vi "LinearBearingControl.vi"() -> ()   [LabVIEW 2012]
uses:
  stressTestTypeDef.ctl
  <vilib>/Utility/error.llb/DialogType.ctl
  allStatesTypeDef.ctl
  <vilib>/Utility/file.llb/Write To Spreadsheet File (DBL).vi
panel:
  out "mm/s (timed)":dbl
  in  "Direction":bool
  in  "Only Move Lin":bool
  out "writing data":bool
  out "stop sys":bool
  out "udp error out":errorcluster
  out "Voltages":dbl[][](array[numeric])
  in  "Start System":bool
  in  "Auto Bias":bool=TRUE
  in  "Unbias":bool
  in  "Bias":bool
  in  "Collect Data":bool=TRUE
  out "Measurement":dbl[][](graph) caption="F/T Data"
  out "Bias Vector":dbl[](array[numeric])
  in  "Timing parameters":T1={"Sample Rate"=1000.0, "Samples to Read"=100}
  in  "Transform":T2
  in  "Channel Parameters":T3={"First Channel"=1, "Number of Channels"=6, "DAQ Card"="Dev2", "Maximum Value"=10.0, "Minimum Value"=-10.0}
  in  "Sensor Parameters":T4={"Calibration File"=path "D:/ArduinoSmarticle/entangledSmarticle/FT21164.cal", "Force Units"="N", "Torque Units"="N-mm"}
  out "filenameOut":string
  in  "Optitrack Parameters":T5={"Optitrack IP"="130.207.141.229", "Optitrack Port"=1520, "timeout (sec)"=80}
  out "Data Output File":path
  in  "Output Folder":path=path "D:/ArduinoSmarticle/entangledSmarticle/Results"
  in  "Program Parameters":T7={"v"=1, "Iters"=2, "Speed"=49, "Delay"=4, "H"=10.5, "SD"=240, "Name"="SS", "Type"=enum."OFF"} {"Speed" min=0 max=49}
  out "strain %":dbl
  out "FT error out":errorcluster
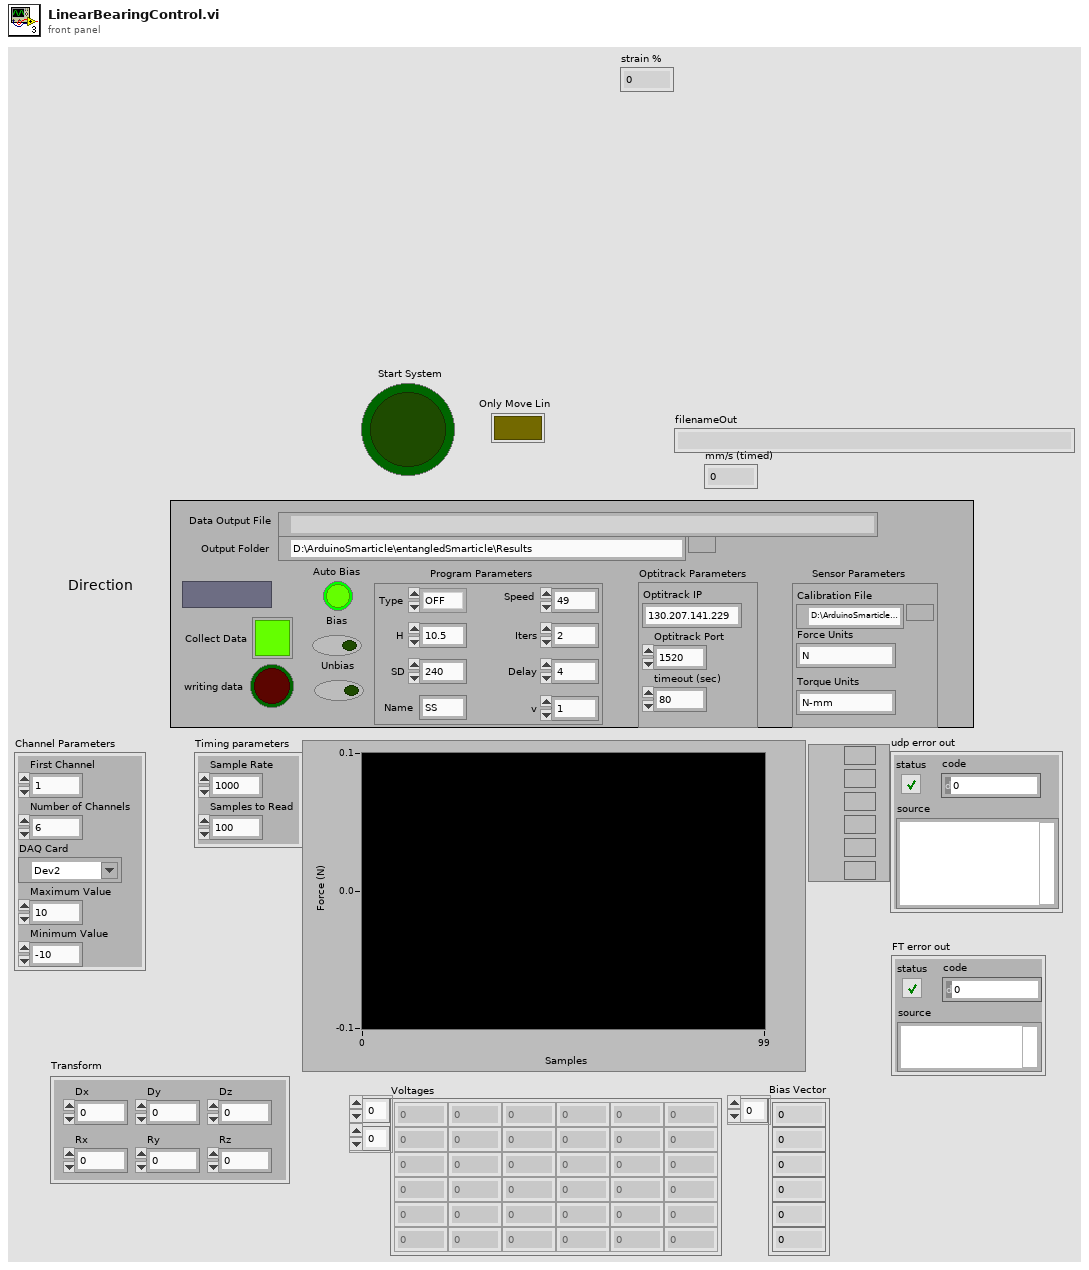
[diagram p1: front panel]
types:
  T1 = cluster{"Sample Rate":dbl, "Samples to Read":i32}
  T2 = cluster{"Dx":dbl, "Dy":dbl, "Dz":dbl, "Rx":dbl, "Ry":dbl, "Rz":dbl}
  T3 = cluster{"First Channel":i16, "Number of Channels":i16, "DAQ Card":tag, "Maximum Value":dbl, "Minimum Value":dbl}
  T4 = cluster{"Calibration File":path, "Force Units":string, "Torque Units":string}
  T5 = cluster{"Optitrack IP":string, "Optitrack Port":u16, "timeout (sec)":i32}
  T6 = typedef "stressTestTypeDef.ctl" = enum16{"OFF", "ON", "EXTEND", "SPRING", "FRACT ON", "SAC", "FRACT SAC"}
  T7 = cluster{"v":i32, "Iters":i32, "Speed":i32, "Delay":i32, "H":dbl, "SD":i32, "Name":string, "Type":T6}
  T8 = typedef "DialogType.ctl" = u16
  T9 = cluster{"SD":i32, "Delay":i32, "Speed":i32, "Iters":i32, "Type":T6}
  T10 = typedef "allStatesTypeDef.ctl" = enum16{"open udp", "start record", "recording", "move linear actuator", "end record", "close udp", "end"}
  T11 = cluster{"distance mm":i32, "Direction":bool, "speed (mm/s)":i32}
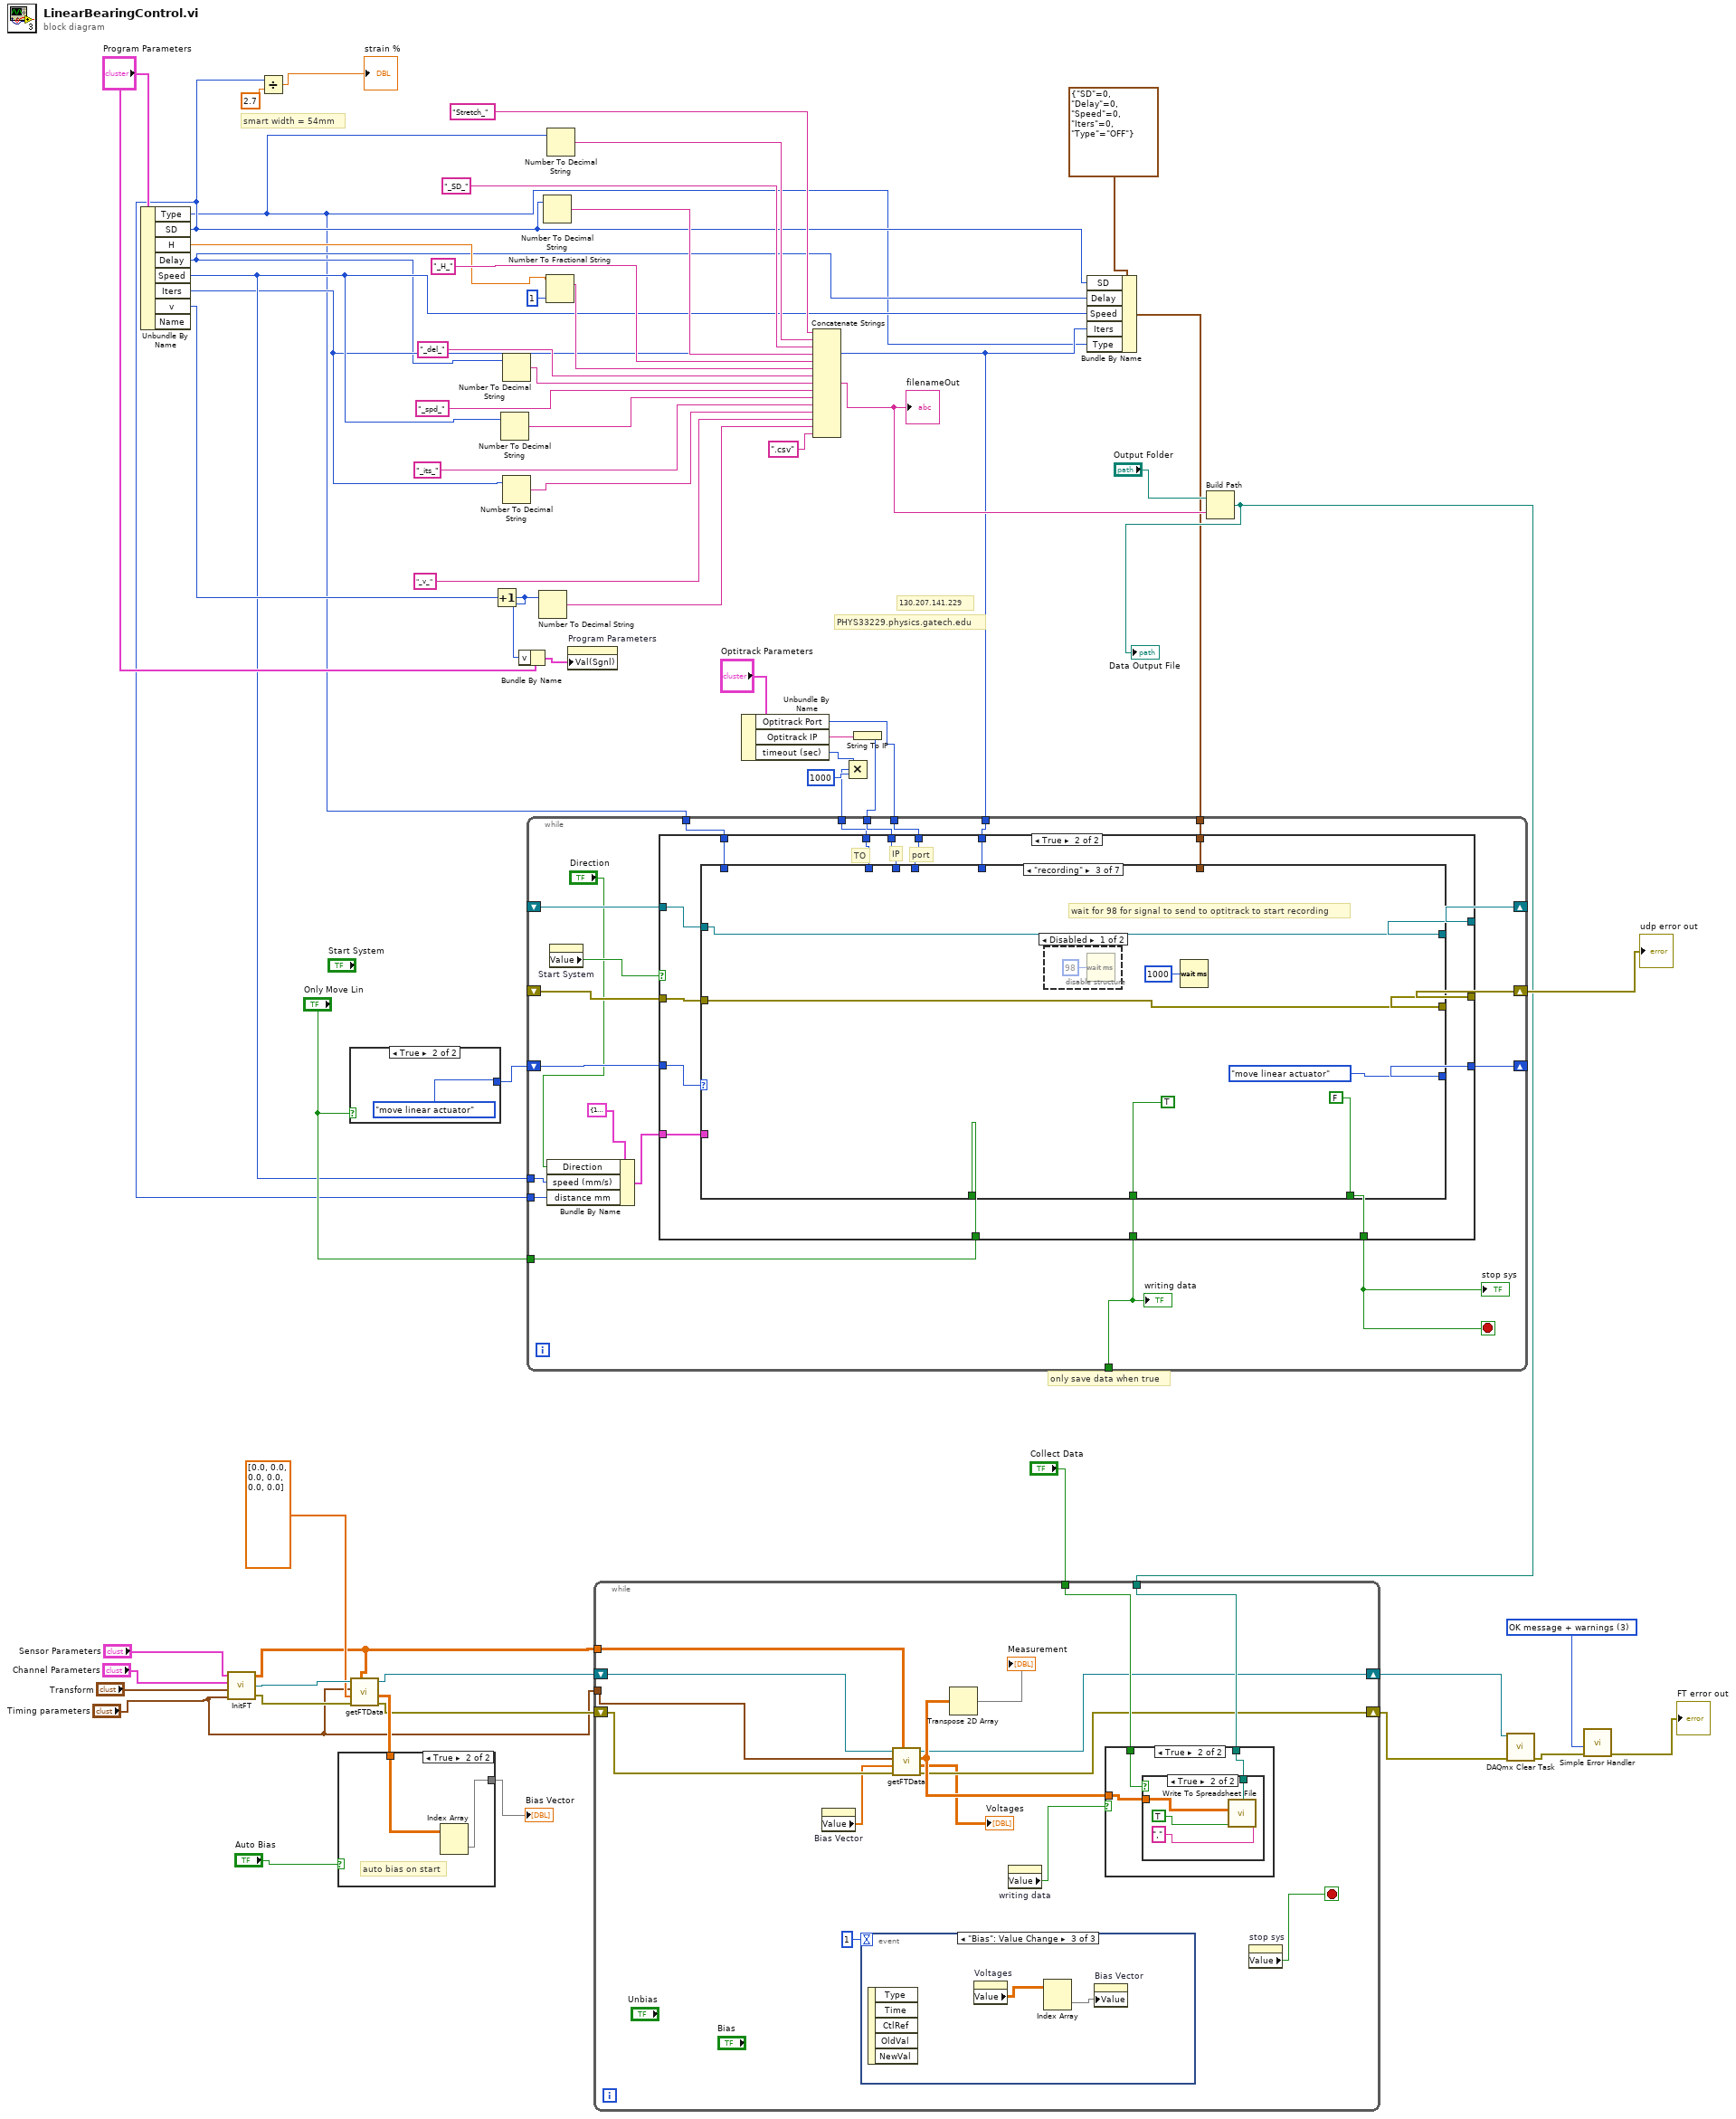
[diagram p0: block diagram]
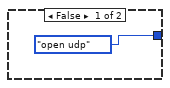
[diagram p2: hidden frame]
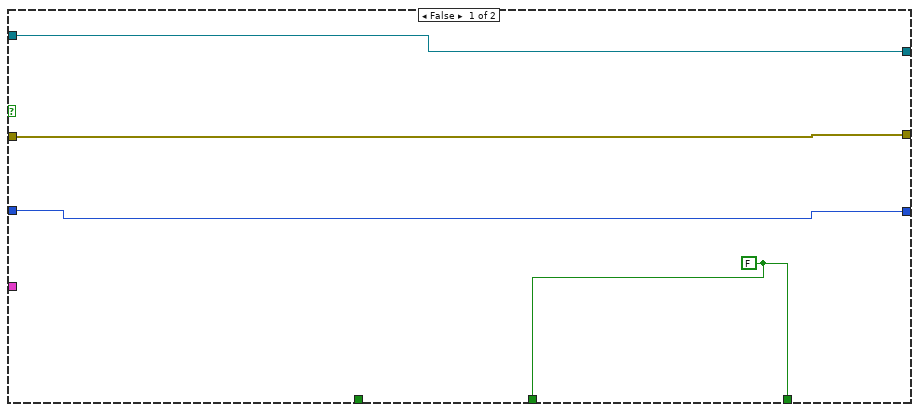
[diagram p3: hidden frame]
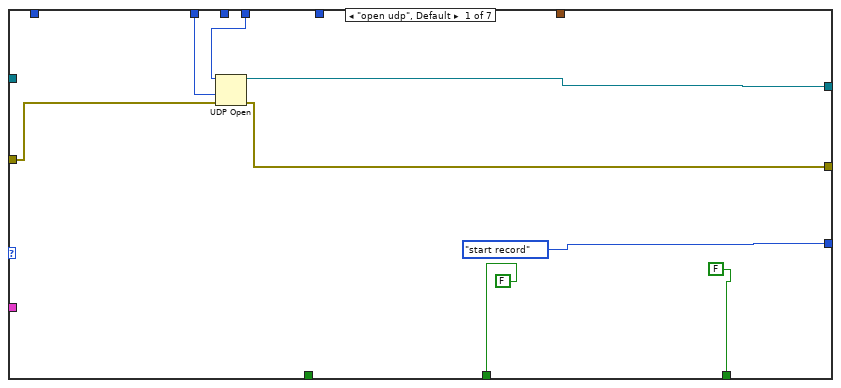
[diagram p4: hidden frame]
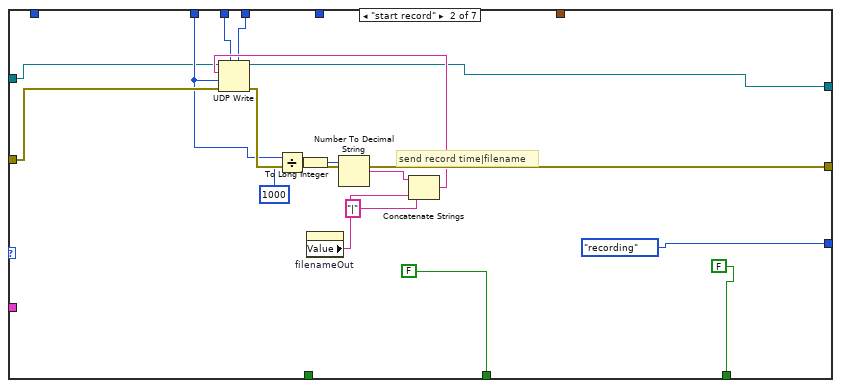
[diagram p5: hidden frame]
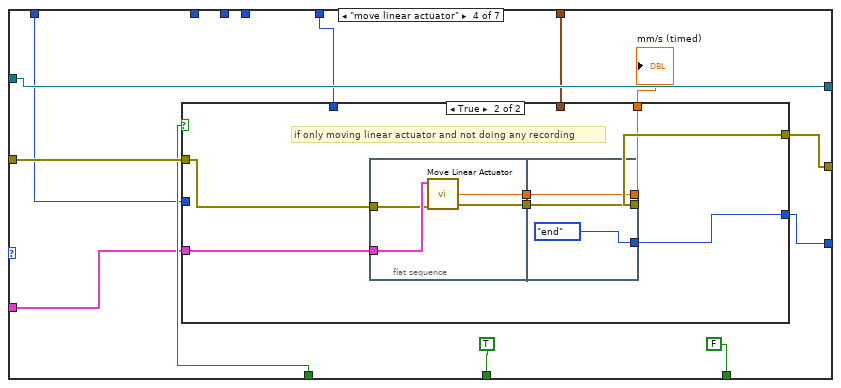
[diagram p7: hidden frame]
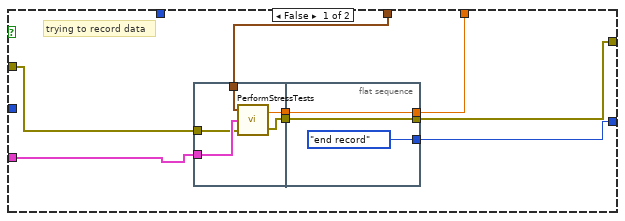
[diagram p8: hidden frame]
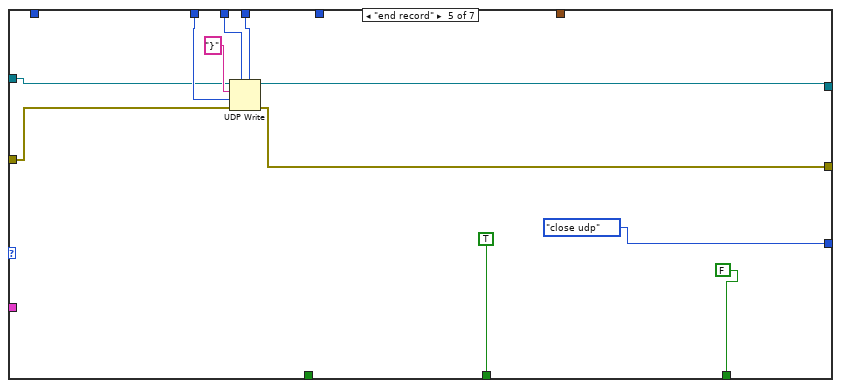
[diagram p9: hidden frame]
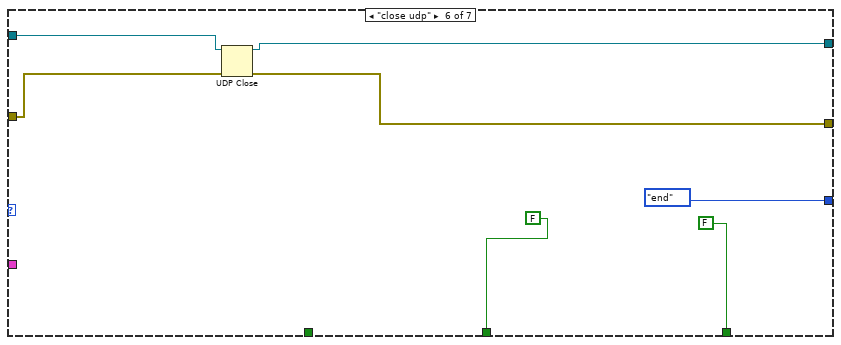
[diagram p10: hidden frame]
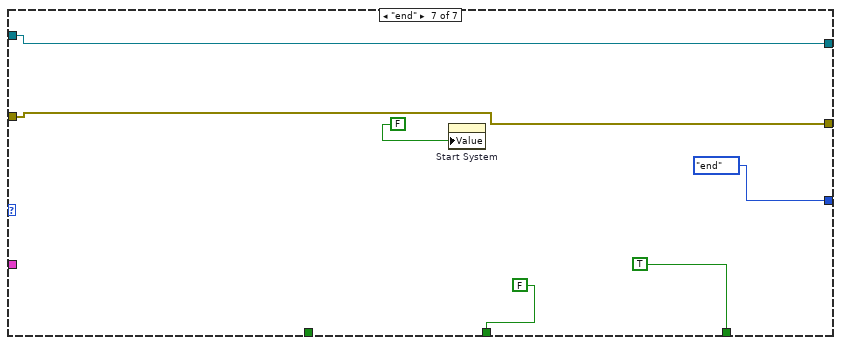
[diagram p11: hidden frame]
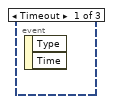
[diagram p12: hidden frame]
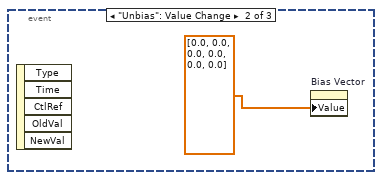
[diagram p13: hidden frame]
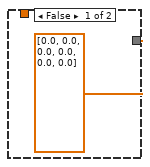
[diagram p16: hidden frame]
diagram:
  w27 = T8 3 items=["no dialog", "OK message", "continue or stop message", "OK message + warnings", "continue/stop + warnings"] ("type of dialog (OK msg:1)")
  # "only save data when true"
  # "smart width = 54mm"
  # "PHYS33229.physics.gatech.edu"
  # "130.207.141.229"
  n1 = Unbundle By Name("Program Parameters") -> ("Type"=w2:T6, "SD"=w5:i32, "H"=w42:dbl, "Delay"=w3:i32, "Speed"=w6:i32, "Iters"=w4:i32, "v"=w43:i32)  [unwired: 1 out]
  n2 = call "InitFT.vi"("Timing parameters"="Timing parameters", "Transform"="Transform", "Channel Parameters"="Channel Parameters", "Sensor Parameters"="Sensor Parameters") -> ("error out"=w23:errorcluster, "task out"=w24:refnum<k21>, "Calibration Matrix"=w18:dbl[][])
  n3 = Divide(x=w5, y=2.7) -> (x/y=→"strain %":dbl)
  n4 = case shown="True" "Only Move Lin" {
    tunnel: [allStatesTypeDef."open udp" allStatesTypeDef."move linear actuator"] -> w62
    frame False {
    }
    frame True {
    }
  }
  n5 = call "getFTData.vi"("Transformed Calibration Matrix"=w18, "error in"=w23, "Bias Vector"=dbl[] [0.0, 0.0, 0.0, 0.0, 0.0, 0.0], "Timing parameters"="Timing parameters", "task in"=w24) -> ("error out"=w16:errorcluster, "Voltages"=w21:dbl[][], "task out 2"=w17:refnum<k21>)  [unwired: 1 out]
  n6 = case shown="True" "Auto Bias" {
    tunnel: w21 -> [_ w67]
    tunnel: [dbl[] [0.0, 0.0, 0.0, 0.0, 0.0, 0.0] w66] -> w14
    frame False {
    }
    frame True {
      # "auto bias on start"
      n7 = Index Array(array=w67) -> (element=w66:dbl[])  [unwired: 2 in]
    }
  }
  "Bias Vector" <- w14
  n8 = Increment(x=w43) -> (x+1=w44:i32)
  n9 = Number To Decimal String(number=w6) -> (decimal integer string=w48:string)  [unwired: 1 in]
  n10 = Number To Decimal String(number=w3) -> (decimal integer string=w54:string)  [unwired: 1 in]
  n11 = Number To Decimal String(number=w4) -> (decimal integer string=w46:string)  [unwired: 1 in]
  n12 = Bundle By Name(cluster="Program Parameters", "v"=w44) -> (w38:T7)
  n13 = Number To Decimal String(number=w44) -> (decimal integer string=w50:string)  [unwired: 1 in]
  n14 = Number To Decimal String(number=w5) -> (decimal integer string=w57:string)  [unwired: 1 in]
  n15 = Number To Fractional String(number=w42, precision (6)=i16 1) -> (F-format string=w53:string)  [unwired: 2 in]
  n16 = Number To Decimal String(number=w2) -> (decimal integer string=w59:string)  [unwired: 1 in]
  n17 = property on="Program Parameters" class="Clust (strict)"("Val(Sgnl)"=w38) -> ()  [unwired: 2 in, 2 out]
  n18 = Unbundle By Name("Optitrack Parameters") -> ("Optitrack Port"=w36:u16, "Optitrack IP"=w35:string, "timeout (sec)"=w33:i32)
  n19 = Concatenate Strings("Stretch_", w59, "_SD_", w57, "_H_", w53, "_del_", w54, "_spd_", w48, "_its_", w46, "_v_", w50, ".csv") -> (w8:string)
  "filenameOut" <- w8
  n20 = Multiply(x=w33, y=1000) -> (x*y=w31:i32)
  n21 = String To IP(1:w35) -> (0:w34:u32)
  n22 = Bundle By Name(cluster=T9 {"SD"=0, "Delay"=0, "Speed"=0, "Iters"=0, "Type"=enum."OFF"}, "SD"=w5, "Delay"=w3, "Speed"=w6, "Iters"=w4, "Type"=w2) -> (w1:T9)
  n23 = while {
    shift-right: [w88] -> w11
    shift-left: _ -> [w87]
    shift-right: [w85] -> _
    shift-left: w62 -> [w86]
    tunnel: w36 -> [w83]
    tunnel: w34 -> [w84]
    tunnel: w31 -> [w82]
    shift-right: [w81] -> _
    shift-left: _ -> [w80]
    tunnel: [w79] -> _
    tunnel: "Only Move Lin" -> [w76]
    tunnel: w6 -> [w73]
    tunnel: w5 -> [w72]
    tunnel: w2 -> [w70]
    tunnel: w4 -> [w69]
    tunnel: w1 -> [w68]
    stop <- w78 stop-if-true
    n24 = Bundle By Name(cluster=T11 {"distance mm"=100, "Direction"=FALSE, "speed (mm/s)"=18} ("linear actuator info"), "Direction"="Direction", "speed (mm/s)"=w73, "distance mm"=w72) -> (w75:T11)
    n25 = property on="Start System" class="Bool (strict)"() -> ("Value"=w77:bool)  [unwired: 2 in, 2 out]
    n26 = case shown="True" w77 {
      tunnel: [w89 w108] -> w88
      tunnel: w87 -> [w89 w107]
      tunnel: w86 -> [w92 w106]
      tunnel: [w92 w105] -> w85
      tunnel: w84 -> [_ w104]
      tunnel: w83 -> [_ w97]
      tunnel: w82 -> [_ w103]
      tunnel: [w90 w102] -> w81
      tunnel: w80 -> [w90 w101]
      tunnel: [w91 w100] -> w79
      tunnel: [w91 w99] -> w78
      tunnel: w76 -> [_ w98]
      tunnel: w75 -> [_ w96]
      tunnel: w70 -> [_ w95]
      tunnel: w69 -> [_ w94]
      tunnel: w68 -> [_ w93]
      frame False {
        w91 = FALSE
      }
      frame True {
        # "IP"
        # "TO"
        # "port"
        n27 = case shown="\"recording\"" w106 {
          tunnel: w103 -> [w113 w125 _ _ w189 _ _]
          tunnel: w107 -> [w114 w131 w135 w148 w193 w199 w201]
          tunnel: [w115 w132 w135 w147 w192 w200 w201] -> w108
          tunnel: [allStatesTypeDef."start record" allStatesTypeDef."recording" allStatesTypeDef."move linear actuator" w150 allStatesTypeDef."close udp" allStatesTypeDef."end" allStatesTypeDef."end"] -> w105
          tunnel: [FALSE FALSE FALSE FALSE FALSE FALSE TRUE] -> w99
          tunnel: w104 -> [_ w118 _ _ w183 _ _]
          tunnel: [w112 w121 w136 w149 w187 w198 w206] -> w102
          tunnel: w101 -> [_ w122 w136 w149 w186 w194 w206]
          tunnel: [FALSE FALSE TRUE TRUE TRUE FALSE FALSE] -> w100
          tunnel: w98 -> [_ _ _ w146 _ _ _]
          tunnel: w97 -> [w109 w117 _ _ w184 _ _]
          tunnel: w96 -> [_ _ _ w145 _ _ _]
          tunnel: w95 -> [_ _ _ w142 _ _ _]
          tunnel: w94 -> [_ _ _ w143 _ _ _]
          tunnel: w93 -> [_ _ _ w141 _ _ _]
          frame "open udp", Default {
            n28 = UDP Open(8:w114, 9:w113, 11:w109) -> (port=w112:refnum<k16>, 0:w115:errorcluster)  [unwired: 2 in, 1 out]
          }
          frame "start record" {
            # "send record time|filename"
            n29 = Divide(x=w125, y=1000) -> (x/y=w124:dbl)
            n30 = To Long Integer(number=w124) -> (32bit integer=w123:i32)
            n31 = property on="filenameOut" class="Str"() -> ("Value"=w129:string)  [unwired: 2 in, 2 out]
            n32 = Number To Decimal String(number=w123) -> (decimal integer string=w127:string)  [unwired: 1 in]
            n33 = Concatenate Strings(w127, "|" ("string"), w129) -> (w128:string)
            n34 = UDP Write(address=w118, port or service name=w117, connection ID=w122, data in=w128, 8:w131, 9:w125) -> (error out=w132:errorcluster, 3:w121:refnum<k16>)
          }
          frame "recording" {
            # "wait for 98 for signal to send to optitrack to start recording"
            n35 = disable-structure shown="Disabled" {
              frame Disabled {
                n36 = Wait (ms)(milliseconds to wait=u32 98) -> ()  [unwired: 1 out]
              }
              frame Enabled {
              }
            }
            n37 = Wait (ms)(milliseconds to wait=u32 1000) -> ()  [unwired: 1 out]
          }
          frame "move linear actuator" {
            n38 = case shown="True" w146 {
              tunnel: [w153 w169] -> w150
              tunnel: w148 -> [w157 w173]
              tunnel: [w156 w174] -> w147
              tunnel: w145 -> [w158 w175]
              tunnel: [w159 w172] -> w144
              tunnel: w143 -> [_ _]
              tunnel: w142 -> [_ _]
              tunnel: w141 -> [w160 _]
              frame False {
                # "trying to record data"
                n39 = flat-sequence {
                  tunnel: w160 -> [w165]
                  tunnel: w158 -> [w163]
                  tunnel: w157 -> [w162]
                  tunnel: [w164] -> w155
                  tunnel: [w161] -> w154
                  tunnel: [w167] -> w156
                  tunnel: [w168] -> w159
                  tunnel: w155 -> [w168]
                  tunnel: w154 -> [w167]
                  tunnel: [allStatesTypeDef."end record"] -> w153
                  frame #0 {
                    n40 = call "PerformStressTests.vi"("error in"=w162, "linear actuator info"=w163, "Test Info"=w165) -> ("error out"=w161:errorcluster, "mm/s (timed)"=w164:dbl)
                  }
                  frame #1 {
                  }
                }
              }
              frame True {
                # "if only moving linear actuator and not doing any recording"
                n41 = flat-sequence {
                  tunnel: w175 -> [w179]
                  tunnel: w173 -> [w177]
                  tunnel: [w178] -> w171
                  tunnel: [w176] -> w170
                  tunnel: [w181] -> w172
                  tunnel: [w182] -> w174
                  tunnel: w171 -> [w182]
                  tunnel: w170 -> [w181]
                  tunnel: [allStatesTypeDef."end"] -> w169
                  frame #0 {
                    n42 = call "Move Linear Actuator.vi"("error in"=w177, "linear actuator info"=w179) -> ("error out"=w178:errorcluster, "mm/s (timed)"=w176:dbl)  [unwired: 2 in, 1 out]
                  }
                  frame #1 {
                  }
                }
              }
            }
            "mm/s (timed)" <- w144
          }
          frame "end record" {
            n43 = UDP Write(address=w183, port or service name=w184, connection ID=w186, data in="}", 8:w193, 9:w189) -> (error out=w192:errorcluster, 3:w187:refnum<k16>)
          }
          frame "close udp" {
            n44 = UDP Close(connection ID=w194, 8:w199) -> (connection ID out=w198:refnum<k16>, error out=w200:errorcluster)
          }
          frame "end" {
            n45 = property on="Start System" class="Bool (strict)"("Value"=FALSE) -> ()  [unwired: 2 in, 2 out]
          }
        }
      }
    }
    "stop sys" <- w78
    "writing data" <- w79
  }
  "udp error out" <- w11
  n46 = Build Path(base path="Output Folder", name or relative path=w8) -> (appended path=w10:path)
  "Data Output File" <- w10
  n47 = while {
    tunnel: w10 -> [w219]
    tunnel: "Collect Data" -> [w218]
    tunnel: w18 -> [w215]
    shift-right: [w217] -> w13
    shift-left: w17 -> [w214]
    shift-right: [w212] -> w12
    shift-left: w16 -> [w216]
    tunnel: "Timing parameters" -> [w213]
    stop <- w208 stop-if-true
    n48 = property on="Bias Vector" class="Arr (strict)"() -> ("Value"=w211:dbl[])  [unwired: 2 in, 2 out]
    n49 = event shown="[2] \"Bias\": Value Change" {
      selector: _ -> [_ _ _]
      dyn-events: _ -> [_ _ _]
      timeout: 1 -> [_ _ _]
      event Timeout {
        n50 = event-data() -> ()  [unwired: 1 in, 2 out]
      }
      event "Unbias": Value Change {
        n51 = event-data() -> ()  [unwired: 1 in, 5 out]
        n52 = property on="Bias Vector" class="Arr (strict)"("Value"=dbl[] [0.0, 0.0, 0.0, 0.0, 0.0, 0.0]) -> ()  [unwired: 2 in, 2 out]
      }
      event "Bias": Value Change {
        n53 = event-data() -> ()  [unwired: 1 in, 5 out]
        n54 = property on="Voltages" class="Arr (strict)"() -> ("Value"=w223:dbl[][])  [unwired: 2 in, 2 out]
        n55 = Index Array(array=w223) -> (element=w224:dbl[])  [unwired: 2 in]
        n56 = property on="Bias Vector" class="Arr (strict)"("Value"=w224) -> ()  [unwired: 2 in, 2 out]
      }
    }
    n57 = call "getFTData.vi"("Transformed Calibration Matrix"=w215, "error in"=w216, "Bias Vector"=w211, "Timing parameters"=w213, "task in"=w214) -> ("error out"=w212:errorcluster, "Voltages"=→"Voltages":dbl[][], "F/T"=w221:dbl[][], "task out 2"=w217:refnum<k21>)
    n58 = Transpose 2D Array(2D array=w221) -> (transposed array=→"Measurement":dbl[][])
    n59 = property on="writing data" class="Bool (strict)"() -> ("Value"=w207:bool)  [unwired: 2 in, 2 out]
    n60 = case shown="True" w207 {
      tunnel: w221 -> [_ w227]
      tunnel: w219 -> [_ w226]
      tunnel: w218 -> [_ w225]
      frame False {
      }
      frame True {
        n61 = case shown="True" w225 {
          tunnel: w227 -> [_ w231]
          tunnel: w226 -> [_ w230]
          frame False {
          }
          frame True {
            n62 = call-poly <vilib>:"Write To Spreadsheet File.vi"("delimiter (\\t)"=",", "append to file? (new file:F)"=TRUE, "2D data"=w231, "file path (dialog if empty)"=w230) -> ()  [unwired: 4 in, 1 out]
          }
        }
      }
    }
    n63 = property on="stop sys" class="Bool (strict)"() -> ("Value"=w208:bool)  [unwired: 2 in, 2 out]
  }
  n64 = call <vilib>:"DAQmx Clear Task.vi"("task in"=w13, "error in"=w12) -> ("error out"=w25:errorcluster)  [unwired: 13 in]
  n65 = call <vilib>:"Simple Error Handler.vi"("type of dialog (OK msg:1)"=w27, "error in (no error)"=w25) -> ("error out"=→"FT error out":errorcluster)  [unwired: 3 in, 4 out]
